vi "scan line.vi"(4 "error in (no error)":errorcluster, 6 "Scan distance":dbl, 8 "Speed":i32, 9 "Min Resolution":dbl format="%#_13g", 10 "Scan Index":i32, 11 "CNC COM in":refnum<visa-resource-name>) -> (1 "error out":errorcluster, 3 "CNC COM out":refnum<visa-resource-name>)   [LabVIEW 2014]
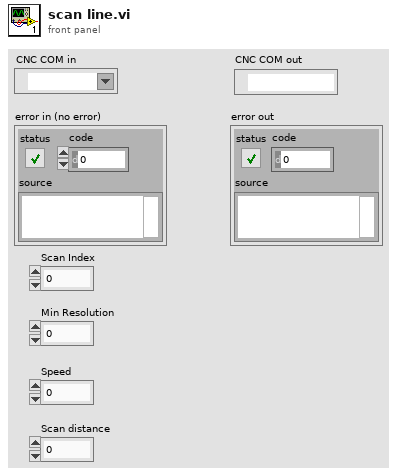
[diagram p1: front panel]
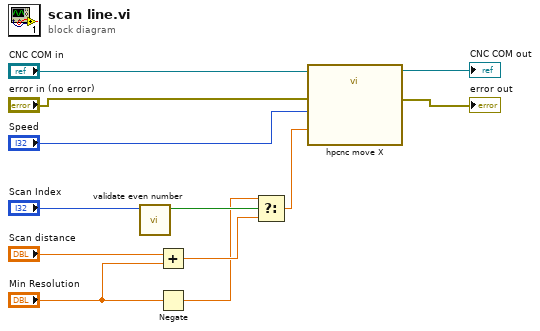
[diagram p0: block diagram]
diagram:
  n1 = call "validate even number.vi"("Number"="Scan Index") -> ("Even"=w7:bool)  [unwired: 10 in]
  n2 = Add(x="Scan distance", y="Min Resolution") -> (x+y=w6:dbl)
  n3 = Negate(x="Min Resolution") -> (-x=w5:dbl)
  n4 = Select(t=w5, s=w7, f=w6) -> (s? t:f=w1:dbl)
  n5 = call "hpcnc move X.vi"("VISA Refnum in"="CNC COM in", "X"=w1, "Speed"="Speed", "error in"="error in (no error)") -> ("VISA Refnum out"=→"CNC COM out":refnum<visa-resource-name>, "error out"=→"error out":errorcluster)  [unwired: 14 in]
